vi "GenerateLogFile.vi"(8 "error in (no error)":errorcluster, 11 "EventFile in":refnum<class "EventFile.lvclass">) -> (0 "error out":errorcluster, 2 "newFile?":bool, 3 "EventFile out":refnum<class "EventFile.lvclass">)   [LabVIEW 2016, in "Event Logging.lvlib" / "EventFile.lvclass"]
uses:
  EventFile.lvclass
  EventFile.lvclass/EventFile.ctl
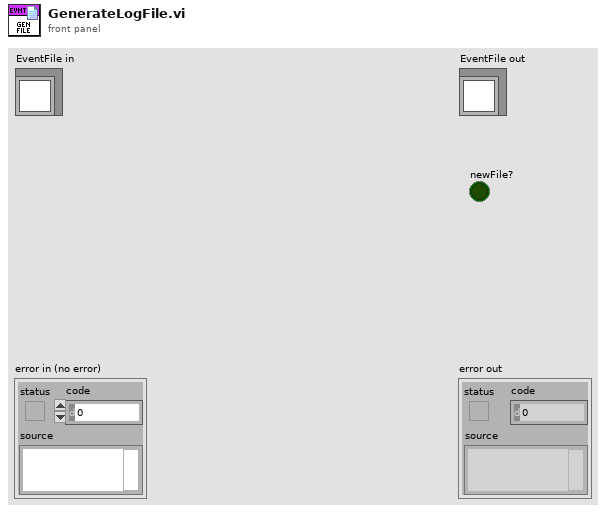
[diagram p1: front panel]
types:
  T1 = enum16{"open", "replace", "create", "open or create", "replace or create", "replace or create with confirmation"}
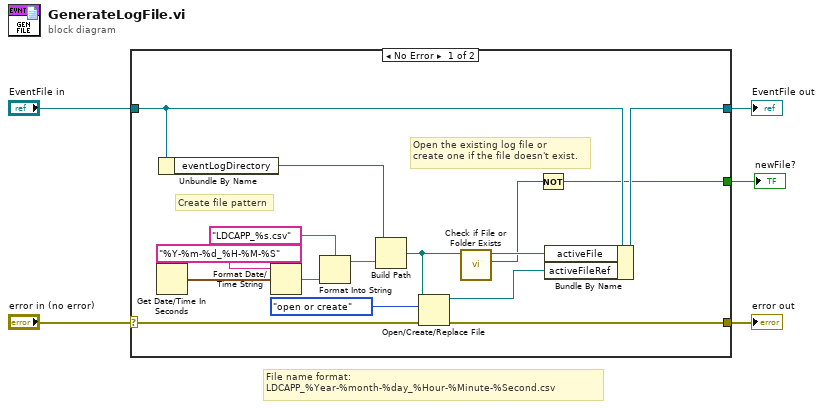
[diagram p0: block diagram]
diagram:
  # "File name format:\nLDCAPP_%Year-%month-%day_%Hour-%Minute-%Second.csv"
  n1 = case shown="No Error" "error in (no error)" {
    selector: "error in (no error)" -> [w14 w23]
    tunnel: [w13 w23] -> w4
    tunnel: [w8 w22] -> w2
    tunnel: "EventFile in" -> [w9 w22]
    tunnel: [w6 _] -> w1
    frame No Error {
      # "Open the existing log file or\ncreate one if the file doesn't exist."
      # "Create file pattern"
      n2 = Get Date/Time In Seconds() -> (seconds since 1Jan1904=w20:timestamp)
      n3 = Unbundle By Name(w9) -> ("eventLogDirectory"=w18:path)
      n4 = Format Date/Time String(time format string (%c)="%Y-%m-%d_%H-%M-%S", seconds (now)=w20) -> (date/time string=w19:string)  [unwired: 1 in]
      n5 = Format Into String(format string="LDCAPP_%s.csv", w19) -> (resulting string=w17:string)  [unwired: 2 in, 1 out]
      n6 = Build Path(base path=w18, name or relative path=w17) -> (appended path=w12:path)
      n7 = Open/Create/Replace File(file path (use dialog)=w12, error in=w14, operation (0:open)=T1."open or create") -> (refnum out=w10:refnum<file>, error out=w13:errorcluster)  [unwired: 3 in, 1 out]
      n8 = call <vilib>:"Check if File or Folder Exists.vi"("path"=w12) -> ("file or folder exists?"=w7:bool, "dup path"=w11:path)  [unwired: 8 in, 1 out]
      n9 = Not(x=w7) -> (.not. x?=w6:bool)
      n10 = Bundle By Name(cluster=w9, "activeFile"=w11, "activeFileRef"=w10) -> (w8:refnum<class "EventFile.lvclass">)
    }
    frame Error {
    }
  }
  "error out" <- w4
  "EventFile out" <- w2
  "newFile?" <- w1
